vi "LOGIN(SubVI).vi"() -> (3 "Boolean":bool)   [LabVIEW 2021]
panel:
  out "OK":bool
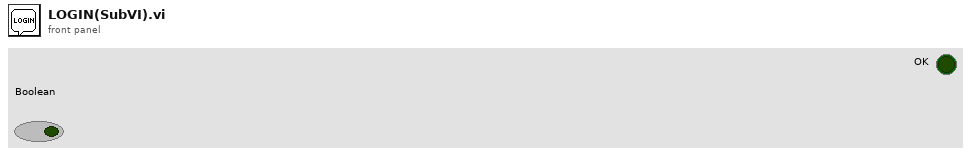
[diagram p1: front panel]
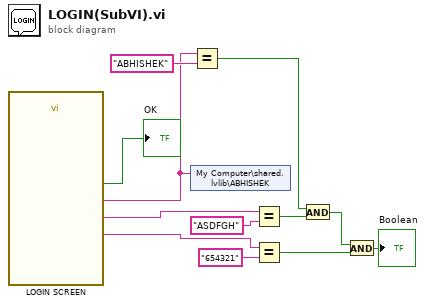
[diagram p0: block diagram]
diagram:
  n1 = call "LOGIN SCREEN"() -> ("ENTER YOUR OTP"=w6:string, "ENTER YOUR PASSWORD"=w4:string, "ENTER YOUR NAME"=w2:string, "OK"=→"OK":bool)  [unwired: 15 in, 1 out]
  n2 = shared-variable "My Computer\\shared.lvlib\\ABHISHEK"(w2) -> ()  [unwired: 1 in, 1 out]
  n3 = Equal?(x=w2, y="ABHISHEK") -> (x = y?=w7:bool)
  n4 = Equal?(x=w4, y="ASDFGH") -> (x = y?=w8:bool)
  n5 = Equal?(x=w6, y="654321") -> (x = y?=w10:bool)
  n6 = And(x=w7, y=w8) -> (x .and. y?=w9:bool)
  n7 = And(x=w9, y=w10) -> (x .and. y?=→"Boolean":bool)
